vi "RX ADU.vi"(8 "error in (no error)":errorcluster, 9 "PDU_req":T1={"Function Code"=1, "Data"=[], "RTU_DataBytes"=0}, 10 "VISA resource in":refnum<visa-resource-name>, 11 "MB_ADU_Serial_RTU in":refnum<class "MB_ADU_RTU.lvclass">) -> (0 "error out":errorcluster, 1 "PDU_resp":T1={"Function Code"=1, "Data"=[], "RTU_DataBytes"=0}, 2 "VISA resource out":refnum<visa-resource-name>, 3 "MB_ADU_Serial_RTU out":refnum<class "MB_ADU_RTU.lvclass">)   [LabVIEW 2016, in "MB Master.lvlib" / "MB_ADU_RTU.lvclass"]
doc: "Defines the receive procedure for a Modbus RTU ADU. The received PDU is written to PDU_resp."
uses:
  MB_ADU_RTU.lvclass
  C:/Users/PRANAV/Downloads/Modbus-Master-master (7)/Modbus-Master-master/MB_ADU/MB_ADU.lvclass
  MB_PDU/MB_PDU_Cluster.ctl
  MB_ADU/MB_ADU.lvclass/MB_ADU.ctl
  MB_ADU/Write RX Timestamp.vi
  MB_ADU/Read Slave ID.vi
  MB_ADU/Write RX Data.vi
  MB Master.lvlib
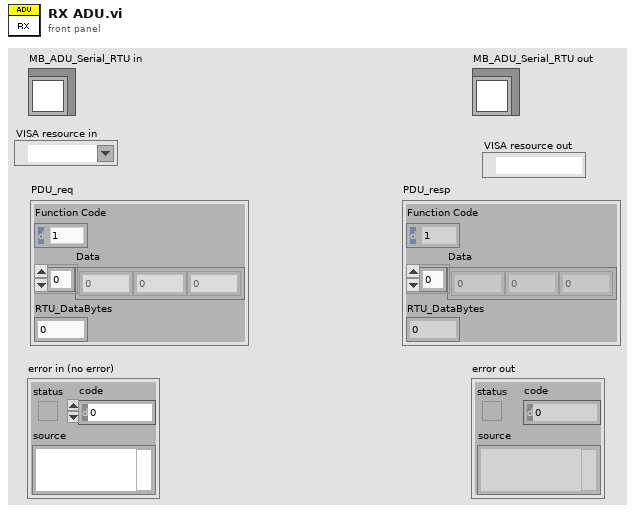
[diagram p1: front panel]
types:
  T1 = typedef "MB Master.lvlib/MB_PDU_Cluster.ctl" = cluster{"Function Code":u8, "Data":u8[], "RTU_DataBytes":i32}
  T2 = enum16{"Read Address", "Read Data", "Read Exception"}
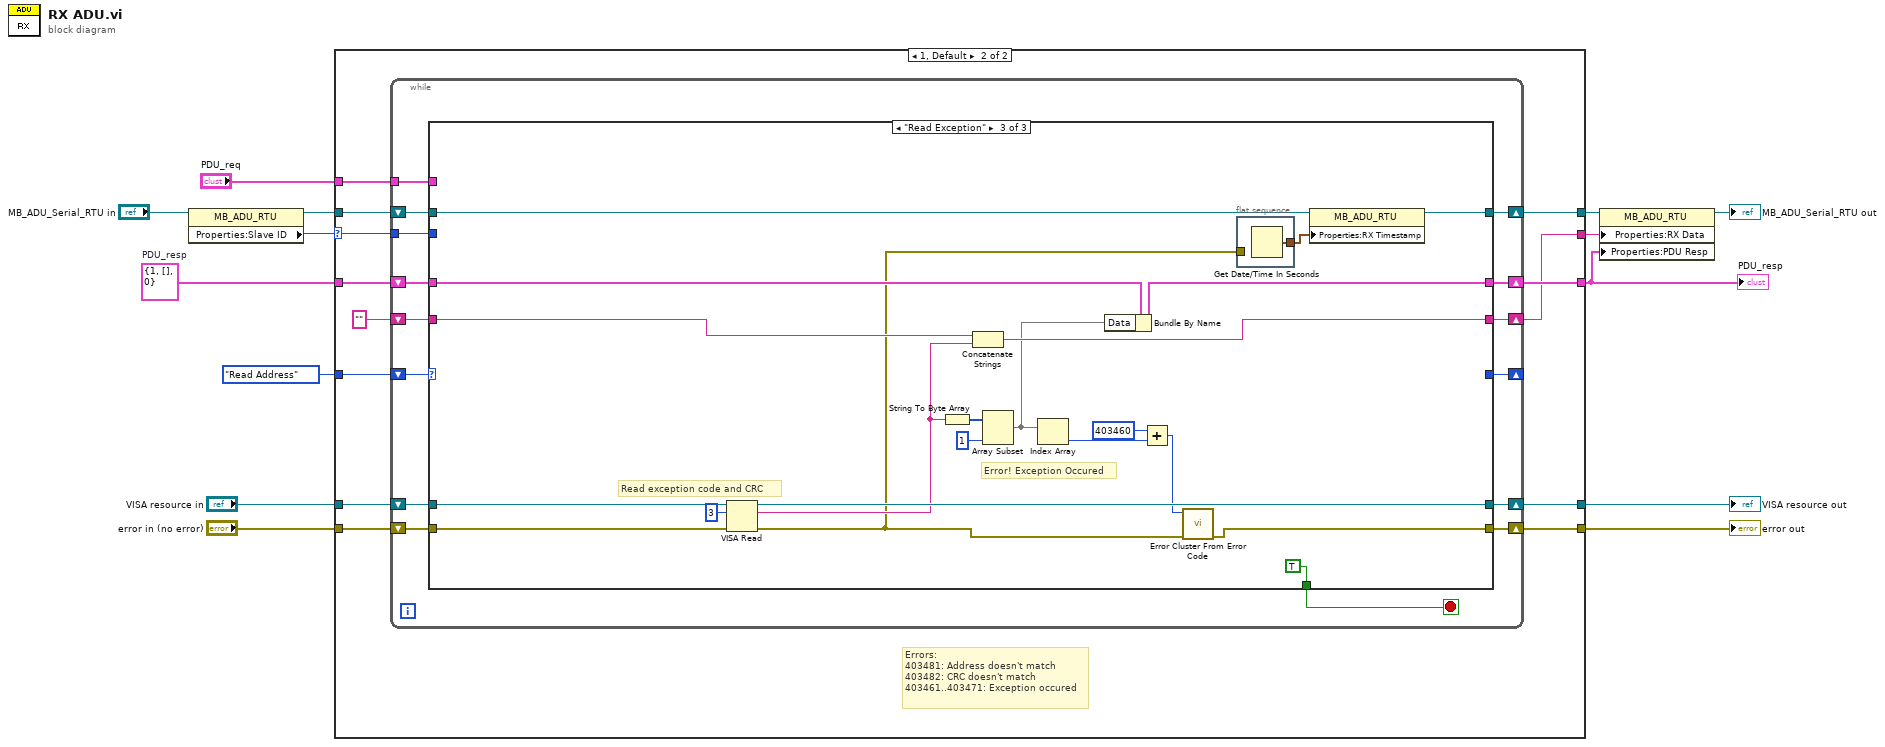
[diagram p0: block diagram]
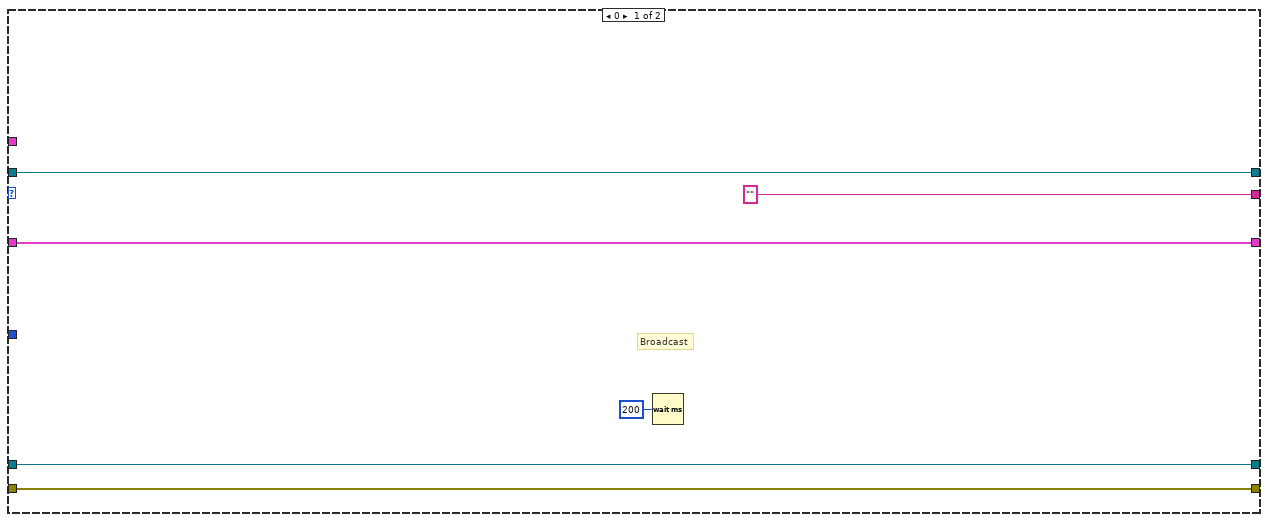
[diagram p2: hidden frame]
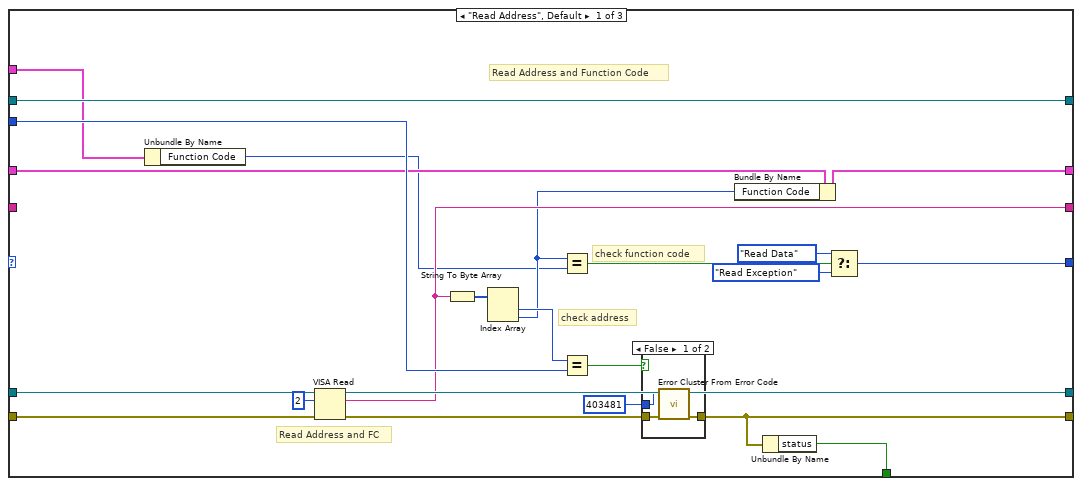
[diagram p3: hidden frame]
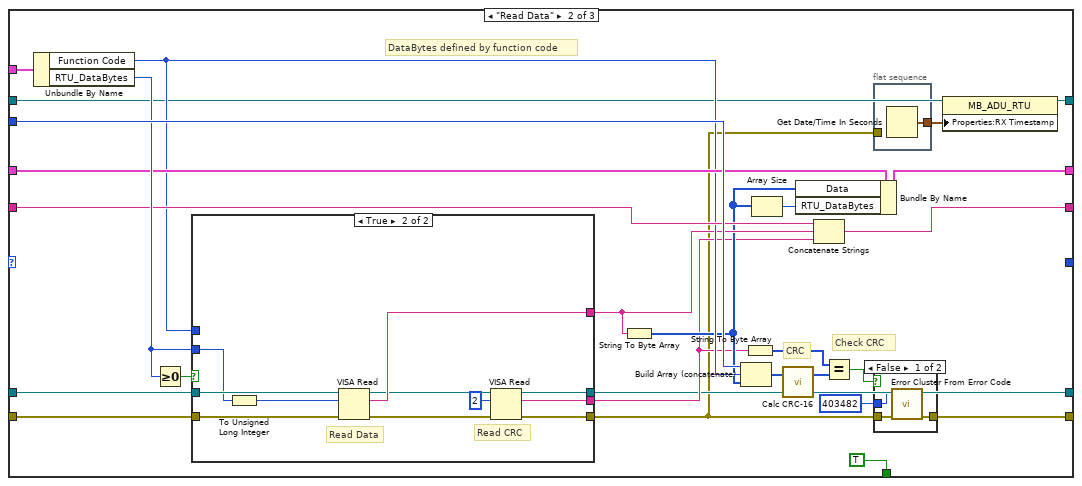
[diagram p5: hidden frame]
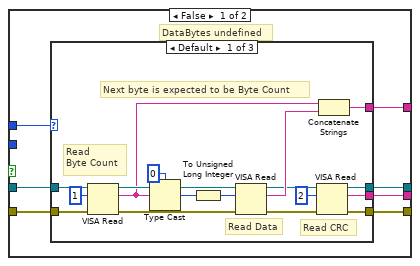
[diagram p7: hidden frame]
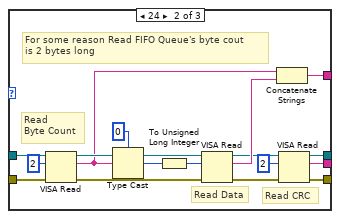
[diagram p8: hidden frame]
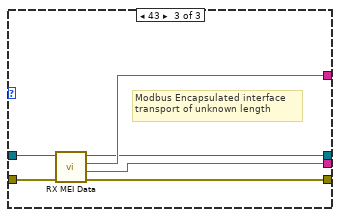
[diagram p9: hidden frame]
diagram:
  w12 = T1 {"Function Code"=1, "Data"=[], "RTU_DataBytes"=0}  # PDU_resp
  n1 = property class="MB_ADU_RTU"(reference="MB_ADU_Serial_RTU in") -> (reference out=w9:refnum<class "MB_ADU_RTU.lvclass">, "Properties:Slave ID"=w4:u8)  [unwired: 1 in, 1 out]
  n2 = case shown="1, Default" w4 {
    selector: w4 -> [_ w23]
    tunnel: "VISA resource in" -> [w17 w33]
    tunnel: "error in (no error)" -> [w16 w32]
    tunnel: w12 -> [w19 w31]
    tunnel: [w19 w30] -> w1
    tunnel: [w17 w29] -> w10
    tunnel: w9 -> [w20 w28]
    tunnel: ["" ("read buffer") w26] -> w8
    tunnel: [w20 w25] -> w7
    tunnel: [w16 w24] -> w6
    tunnel: "PDU_req" -> [_ w21]
    tunnel: T2."Read Address" -> [_ w22]
    frame 0 {
      # "Broadcast"
      n3 = Wait (ms)(milliseconds to wait=u32 200) -> ()  [unwired: 1 out]
    }
    frame 1, Default {
      # "Errors:\n403481: Address doesn't match\n403482: CRC doesn't match\n403461..403471: Exception occured"
      n4 = while {
        shift-right: [w46] -> w29
        shift-left: w33 -> [w47]
        shift-right: [w36] -> w24
        shift-left: w32 -> [w45]
        shift-right: [w37] -> _
        shift-left: w22 -> [w48]
        shift-right: [w43] -> w30
        shift-left: w31 -> [w44]
        tunnel: w23 -> [w42]
        shift-right: [w38] -> w25
        shift-left: w28 -> [w41]
        shift-right: [w40] -> w26
        shift-left: "" ("read buffer") -> [w39]
        tunnel: w21 -> [w34]
        stop <- w35 stop-if-true
        n5 = case shown="\"Read Exception\"" w48 {
          tunnel: w47 -> [w68 w102 w186]
          tunnel: [w71 w77 w183] -> w46
          tunnel: w45 -> [w69 w101 w185]
          tunnel: [w59 _ _] -> w37
          tunnel: [w54 w92 w167] -> w36
          tunnel: [w55 TRUE TRUE] -> w35
          tunnel: w44 -> [w53 w86 w182]
          tunnel: [w51 w96 w181] -> w43
          tunnel: w42 -> [w65 w90 _]
          tunnel: w41 -> [w63 w79 w176]
          tunnel: [w62 w87 w178] -> w40
          tunnel: w39 -> [_ w85 w180]
          tunnel: [w63 w100 w175] -> w38
          tunnel: w34 -> [w49 w88 _]
          frame "Read Address", Default {
            # "check function code"
            # "check address"
            # "Read Address and FC"
            # "Read Address and Function Code"
            n6 = Unbundle By Name(w49) -> ("Function Code"=w50:u8)
            n7 = VISA Read(VISA resource name=w68, byte count=u32 2, error in (no error)=w69) -> (VISA resource name out=w71:refnum<visa-resource-name>, read buffer=w62:string, error out=w67:errorcluster)  [unwired: 1 out]
            n8 = String To Byte Array(string=w62) -> (unsigned byte array=w61:u8[])
            n9 = Index Array(array=w61) -> (element #1=w60:u8, element #2=w52:u8)  [unwired: 2 in]
            n10 = Equal?(x=w52, y=w50) -> (x = y?=w58:bool)
            n11 = Equal?(x=w60, y=w65) -> (x = y?=w64:bool)
            n12 = case shown="False" w64 {
              tunnel: [w73 w75] -> w54
              tunnel: w67 -> [w74 w75]
              tunnel: 403481 ("error code (0)") -> [w72 _]
              frame False {
                n13 = call <vilib>:"Error Cluster From Error Code.vi"("error in (no error)"=w74, "error code (0)"=w72) -> ("error out"=w73:errorcluster)  [unwired: 7 in]
              }
              frame True {
              }
            }
            n14 = Bundle By Name(cluster=w53, "Function Code"=w52) -> (w51:T1)
            n15 = Unbundle By Name(w54) -> ("status"=w55:bool)
            n16 = Select(t=T2."Read Data", s=w58, f=T2."Read Exception") -> (s? t:f=w59:T2)
          }
          frame "Read Data" {
            # "CRC"
            # "Check CRC"
            # "DataBytes defined by function code"
            n17 = Unbundle By Name(w88) -> ("Function Code"=w84:u8, "RTU_DataBytes"=w89:i32)
            n18 = Greater Or Equal To 0?(x=w89) -> (x >= 0?=w97:bool)
            n19 = case shown="True" w97 {
              tunnel: w102 -> [w114 w165]
              tunnel: w101 -> [w113 w164]
              tunnel: [w112 w157] -> w77
              tunnel: [w111 w156] -> w76
              tunnel: w89 -> [_ w161]
              tunnel: [w110 w163] -> w82
              tunnel: w84 -> [w109 _]
              tunnel: [w108 w155] -> w78
              frame False {
                # "DataBytes undefined"
                n20 = case shown="Default" w109 {
                  tunnel: w114 -> [w131 w148 w154]
                  tunnel: w113 -> [w130 w147 w153]
                  tunnel: [w119 w136 w151] -> w112
                  tunnel: [w118 w135 w150] -> w111
                  tunnel: [w123 w142 w152] -> w110
                  tunnel: [w117 w134 w149] -> w108
                  frame Default {
                    # "Read CRC"
                    # "Read Data"
                    # "Read\nByte Count"
                    # "Next byte is expected to be Byte Count"
                    n21 = VISA Read(VISA resource name=w131, byte count=u32 1, error in (no error)=w130) -> (VISA resource name out=w127:refnum<visa-resource-name>, read buffer=w125:string, error out=w126:errorcluster)  [unwired: 1 out]
                    n22 = Type Cast(type=u8 0, x=w125) -> (*(type *) &x=w122:u8)
                    n23 = To Unsigned Long Integer(number=w122) -> (unsigned 32bit integer=w121:u32)
                    n24 = VISA Read(VISA resource name=w127, byte count=w121, error in (no error)=w126) -> (VISA resource name out=w116:refnum<visa-resource-name>, read buffer=w124:string, error out=w115:errorcluster)  [unwired: 1 out]
                    n25 = VISA Read(VISA resource name=w116, byte count=u32 2, error in (no error)=w115) -> (VISA resource name out=w119:refnum<visa-resource-name>, read buffer=w117:string, error out=w118:errorcluster)  [unwired: 1 out]
                    n26 = Concatenate Strings(w125, w124) -> (w123:string)
                  }
                  frame 24 {
                    # "Read CRC"
                    # "Read Data"
                    # "Read\nByte Count"
                    # "For some reason Read FIFO Queue's byte cout\nis 2 bytes long"
                    n27 = VISA Read(VISA resource name=w148, byte count=u32 2, error in (no error)=w147) -> (VISA resource name out=w145:refnum<visa-resource-name>, read buffer=w140:string, error out=w144:errorcluster)  [unwired: 1 out]
                    n28 = Type Cast(type=u16 0, x=w140) -> (*(type *) &x=w138:u16)
                    n29 = To Unsigned Long Integer(number=w138) -> (unsigned 32bit integer=w139:u32)
                    n30 = VISA Read(VISA resource name=w145, byte count=w139, error in (no error)=w144) -> (VISA resource name out=w133:refnum<visa-resource-name>, read buffer=w143:string, error out=w132:errorcluster)  [unwired: 1 out]
                    n31 = Concatenate Strings(w140, w143) -> (w142:string)
                    n32 = VISA Read(VISA resource name=w133, byte count=u32 2, error in (no error)=w132) -> (VISA resource name out=w136:refnum<visa-resource-name>, read buffer=w134:string, error out=w135:errorcluster)  [unwired: 1 out]
                  }
                  frame 43 {
                    # "Modbus Encapsulated interface\ntransport of unknown length"
                    n33 = call "RX MEI Data.vi"("error in (no error)"=w153, "VISA resource in"=w154) -> ("error out"=w150:errorcluster, "CRC"=w149:string, "Data Buffer"=w152:string, "VISA resource out"=w151:refnum<visa-resource-name>)  [unwired: 6 in]
                  }
                }
              }
              frame True {
                # "Read CRC"
                # "Read Data"
                n34 = To Unsigned Long Integer(number=w161) -> (unsigned 32bit integer=w162:u32)
                n35 = VISA Read(VISA resource name=w165, byte count=w162, error in (no error)=w164) -> (VISA resource name out=w159:refnum<visa-resource-name>, read buffer=w163:string, error out=w158:errorcluster)  [unwired: 1 out]
                n36 = VISA Read(VISA resource name=w159, byte count=u32 2, error in (no error)=w158) -> (VISA resource name out=w157:refnum<visa-resource-name>, read buffer=w155:string, error out=w156:errorcluster)  [unwired: 1 out]
              }
            }
            n37 = String To Byte Array(string=w82) -> (unsigned byte array=w80:u8[])
            n38 = Build Array (concatenate)(w90, w84, w80) -> (w91:u8[])
            n39 = String To Byte Array(string=w78) -> (unsigned byte array=w83:u8[])
            n40 = Array Size(array=w80) -> (size(s)=w81:i32)
            n41 = call "Calc CRC-16.vi"("Frame in"=w91) -> ("CRC-16"=w93:u8[])  [unwired: 2 in]
            n42 = Bundle By Name(cluster=w86, "Data"=w80, "RTU_DataBytes"=w81) -> (w96:T1)
            n43 = Concatenate Strings(w85, w82, w78) -> (w87:string)
            n44 = Equal?(x=w83, y=w93) -> (x = y?=w95:bool)
            n45 = flat-sequence {
              tunnel: [w103] -> w99
              tunnel: w76 -> [_]
              frame #0 {
                n46 = Get Date/Time In Seconds() -> (seconds since 1Jan1904=w103:timestamp)
              }
            }
            n47 = case shown="False" w95 {
              tunnel: [w105 w107] -> w92
              tunnel: w76 -> [w106 w107]
              tunnel: 403482 ("error code (0)") -> [w104 _]
              frame False {
                n48 = call <vilib>:"Error Cluster From Error Code.vi"("error in (no error)"=w106, "error code (0)"=w104) -> ("error out"=w105:errorcluster)  [unwired: 7 in]
              }
              frame True {
              }
            }
            n49 = property class="MB_ADU_RTU"(reference=w79, "Properties:RX Timestamp"=w99) -> (reference out=w100:refnum<class "MB_ADU_RTU.lvclass">)  [unwired: 1 in, 1 out]
          }
          frame "Read Exception" {
            # "Error! Exception Occured"
            # "Read exception code and CRC"
            n50 = VISA Read(VISA resource name=w186, byte count=u32 3, error in (no error)=w185) -> (VISA resource name out=w183:refnum<visa-resource-name>, read buffer=w179:string, error out=w166:errorcluster)  [unwired: 1 out]
            n51 = String To Byte Array(string=w179) -> (unsigned byte array=w169:u8[])
            n52 = Concatenate Strings(w180, w179) -> (w178:string)
            n53 = Array Subset(array=w169, length=1) -> (w168:u8[])  [unwired: 1 in]
            n54 = Index Array(array=w168) -> (element=w171:u8)  [unwired: 1 in]
            n55 = Bundle By Name(cluster=w182, "Data"=w168) -> (w181:T1)
            n56 = Add(x=403460 ("error code (0)"), y=w171) -> (x+y=w170:i32)
            n57 = call <vilib>:"Error Cluster From Error Code.vi"("error in (no error)"=w166, "error code (0)"=w170) -> ("error out"=w167:errorcluster)  [unwired: 7 in]
            n58 = flat-sequence {
              tunnel: [w187] -> w174
              tunnel: w166 -> [_]
              frame #0 {
                n59 = Get Date/Time In Seconds() -> (seconds since 1Jan1904=w187:timestamp)
              }
            }
            n60 = property class="MB_ADU_RTU"(reference=w176, "Properties:RX Timestamp"=w174) -> (reference out=w175:refnum<class "MB_ADU_RTU.lvclass">)  [unwired: 1 in, 1 out]
          }
        }
      }
    }
  }
  "error out" <- w6
  "VISA resource out" <- w10
  "PDU_resp" <- w1
  n61 = property class="MB_ADU_RTU"(reference=w7, "Properties:RX Data"=w8, "Properties:PDU Resp"=w1) -> (reference out=→"MB_ADU_Serial_RTU out":refnum<class "MB_ADU_RTU.lvclass">)  [unwired: 1 in, 1 out]
